vi "Acquire PWM.vi"(11 "Bank in":refnum<class "Bank.lvclass">) -> (1 "Connector <m> Bank <n>":T1, 3 "Bank out":refnum<class "Bank.lvclass">)   [LabVIEW 2019, in "LRUTS FPGA IP.lvlib" / "Bank.lvclass"]
uses:
  source/Bank/Bank.lvclass
  <instrlib>/_niInstr/Basic Elements/v1/FPGA/niInstr Basic Elements v1 FPGA.lvlib
  source/Bank/Bank Type.ctl
  <vilib>/eio/EIONode/EIONode.xnode
  source/Bank/Discrete Acquisition Bank.ctl
  <vilib>/rvi/eio/common/nirviEmuTemplateMethod_errors.vi
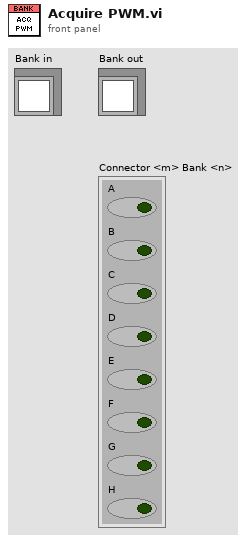
[diagram p1: front panel]
types:
  T1 = typedef "LRUTS FPGA IP.lvlib/Bank.lvclass/Discrete Acquisition Bank.ctl" = cluster{"A":bool, "B":bool, "C":bool, "D":bool, "E":bool, "F":bool, "G":bool, "H":bool}
  T2 = typedef "LRUTS FPGA IP.lvlib/Bank.lvclass/Bank Type.ctl" = enum16{"None", "Discrete Acquisition", "Discrete Generation", "PWM Acquisition", "PWM Generation"}
  T3 = typedef "LRUTS FPGA IP.lvlib/Bank.lvclass/DIO Resources.ctl" = cluster{"DIO 0":refnum<k21>, "DIO 1":refnum<k21>, "DIO 2":refnum<k21>, "DIO 3":refnum<k21>, "DIO 4":refnum<k21>, "DIO 5":refnum<k21>, "DIO 6":refnum<k21>, "DIO 7":refnum<k21>}
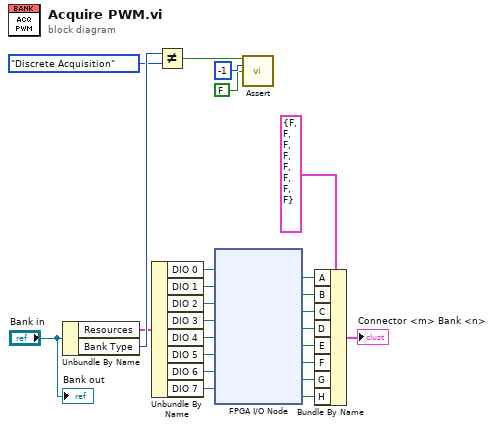
[diagram p0: block diagram]
diagram:
  n1 = Unbundle By Name("Bank in") -> ("Resources"=w19:T3, "Bank Type"=w24:T2)
  n2 = Unbundle By Name(w19) -> ("DIO 0"=w18:refnum<k21>, "DIO 1"=w17:refnum<k21>, "DIO 2"=w16:refnum<k21>, "DIO 3"=w15:refnum<k21>, "DIO 4"=w14:refnum<k21>, "DIO 5"=w13:refnum<k21>, "DIO 6"=w12:refnum<k21>, "DIO 7"=w11:refnum<k21>)
  n3 = Not Equal?(x=w24, y=Bank_Type."Discrete Acquisition") -> (x != y?=w22:bool)
  n4 = xnode "FPGA I/O Node"("FPGA I/O In"=w18, "FPGA I/O In"=w17, "FPGA I/O In"=w16, "FPGA I/O In"=w15, "FPGA I/O In"=w14, "FPGA I/O In"=w13, "FPGA I/O In"=w12, "FPGA I/O In"=w11) -> ("I/O Item"=w8:bool, "I/O Item"=w7:bool, "I/O Item"=w6:bool, "I/O Item"=w5:bool, "I/O Item"=w4:bool, "I/O Item"=w3:bool, "I/O Item"=w2:bool, "I/O Item"=w1:bool)  [unwired: 8 out]
  n5 = call <instrlib>:"Assert.vi"("assert"=w22, "error code"=-1, "enable show error"=FALSE) -> ()  [unwired: 13 in]
  n6 = Bundle By Name(cluster=T1 {"A"=FALSE, "B"=FALSE, "C"=FALSE, "D"=FALSE, "E"=FALSE, "F"=FALSE, "G"=FALSE, "H"=FALSE} ("Connector <m> Bank <n>"), "A"=w8, "B"=w7, "C"=w6, "D"=w5, "E"=w4, "F"=w3, "G"=w2, "H"=w1) -> (→"Connector <m> Bank <n>":T1)
  "Bank out" <- "Bank in"
